vi "Select Hardware.vi"(8 "error in (no error)":errorcluster, 10 "Hardware":T4(ring), 11 "File INI.Hardware DAQ":T3) -> (0 "error out":errorcluster, 2 "#Parametros HW":T2, 3 "Reference HW":T1)   [LabVIEW 2020, in "Hardware DAQ.lvlib"]
uses:
  Hardware DAQ.lvlib
  <vilib>/Modbus/master/Modbus Master.lvclass
  <vilib>/Instr/_visa.llb/VISA Configure Serial Port (Instr).vi
  <vilib>/Modbus/master/Create Master Instance (TCP).vi
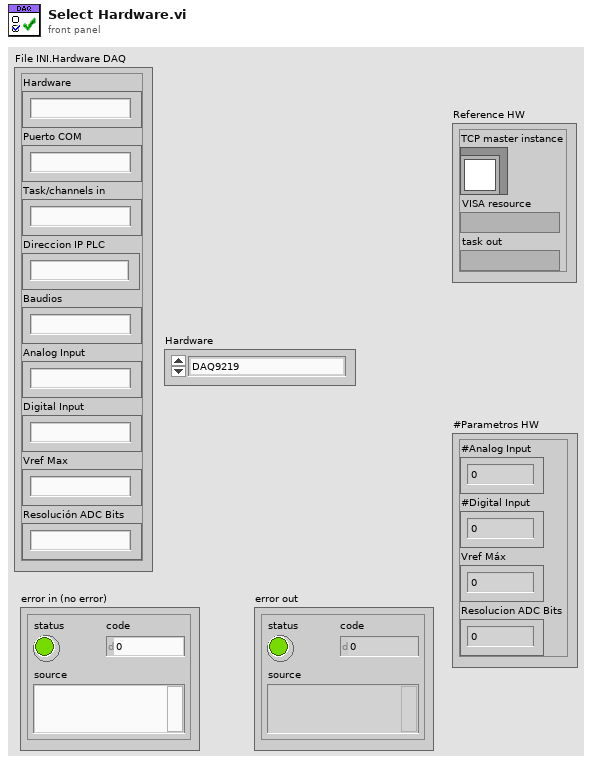
[diagram p1: front panel]
types:
  T1 = cluster{"TCP master instance":refnum<class "Modbus Master.lvclass">, "VISA resource":refnum<visa-resource-name>, "task out":refnum<k21>}
  T2 = cluster{"#Analog Input":i32, "#Digital Input":i32, "Vref Máx":i32, "Resolucion ADC Bits":i32}
  T3 = cluster{"Hardware":string, "Puerto COM":string, "Task/channels in":string, "Direccion IP PLC":string, "Baudios":string, "Analog Input":string, "Digital Input":string, "Vref Max":string, "Resolución ADC Bits":string}
  T4 = enum16{"DAQ9219", "Arduino", "Xpress Board", "PLC Logo", "Default"}
  T5 = cluster{"TCP master instance":refnum<class "Modbus Master.lvclass">, "VISA resource name out":refnum<visa-resource-name>, "task out":refnum<k21>}
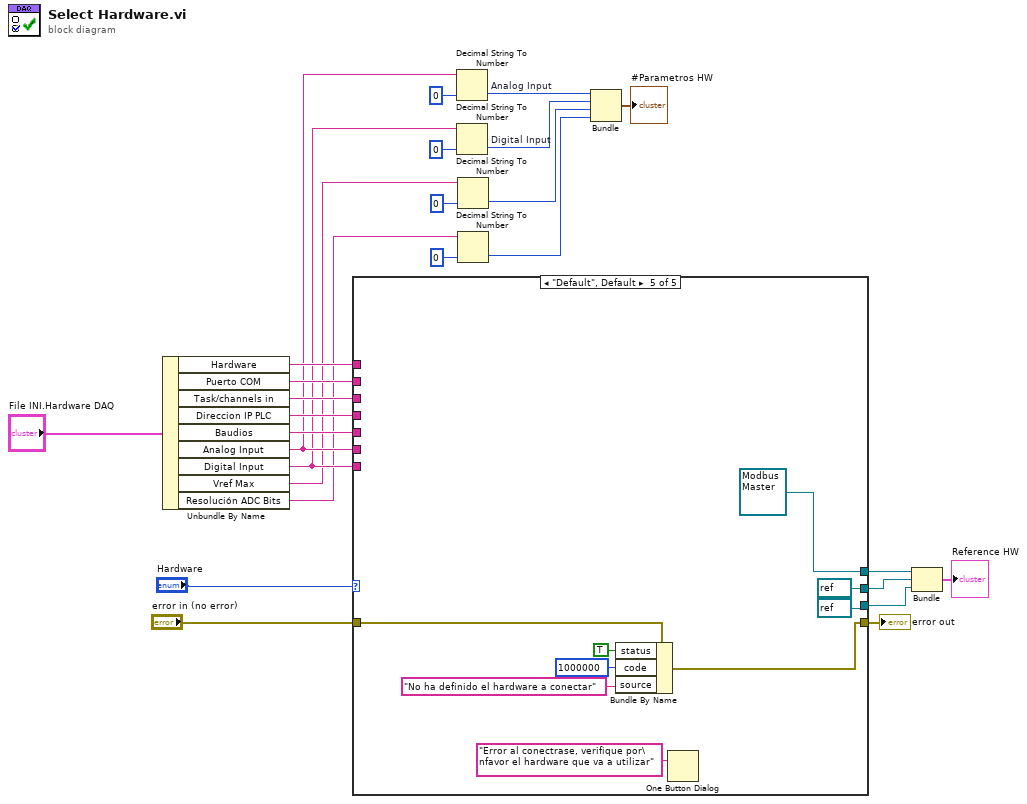
[diagram p0: block diagram]
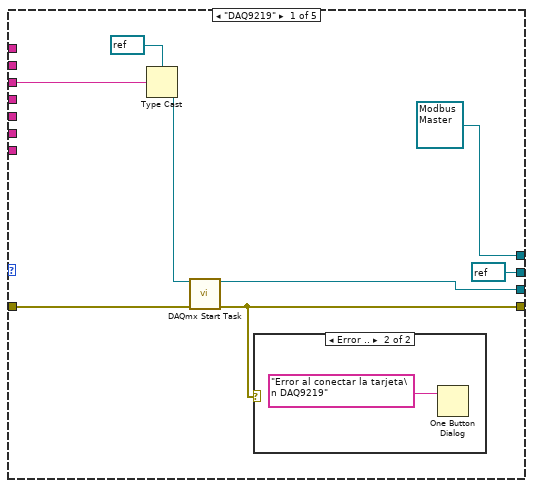
[diagram p2: hidden frame]
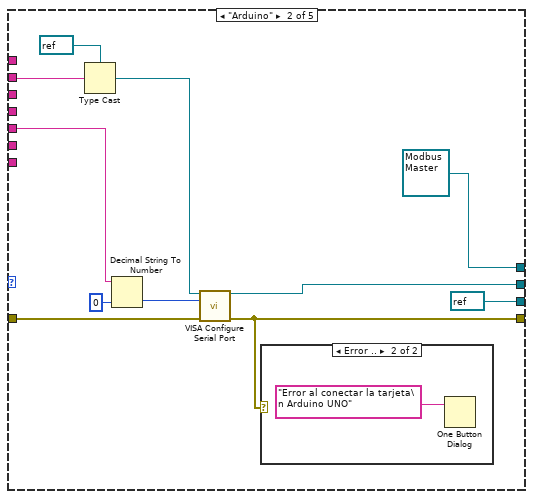
[diagram p4: hidden frame]
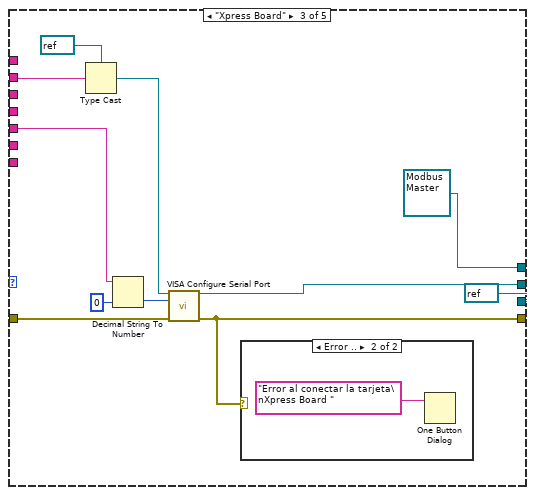
[diagram p6: hidden frame]
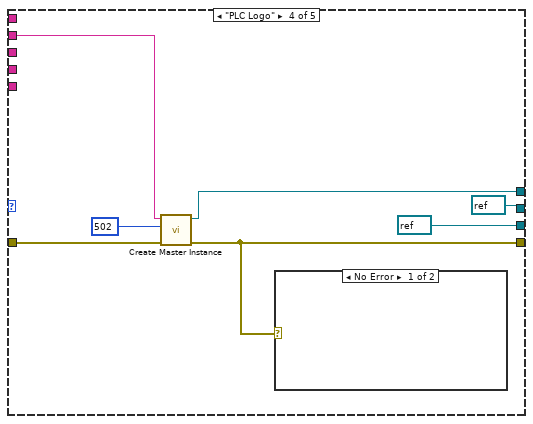
[diagram p8: hidden frame]
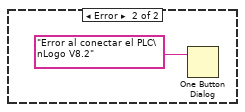
[diagram p9: hidden frame]
diagram:
  n1 = Unbundle By Name("File INI.Hardware DAQ") -> ("Hardware"=w20:string, "Puerto COM"=w21:string, "Task/channels in"=w24:string, "Direccion IP PLC"=w23:string, "Baudios"=w22:string, "Analog Input"=w19:string, "Digital Input"=w16:string, "Vref Max"=w11:string, "Resolución ADC Bits"=w10:string)
  n2 = case shown="\"Default\", Default" "Hardware" {
    tunnel: "error in (no error)" -> [w32 w44 w55 w65 w72]
    tunnel: [w27 w36 w48 w60 w70] -> w26
    tunnel: w21 -> [_ w37 w57 _ _]
    tunnel: [w31 refnum<k21> refnum ("task out") refnum<k21> refnum ("task out") refnum<k21> refnum ("task out") refnum<k21> refnum ("task out")] -> w2
    tunnel: [refnum<visa-resource-name> refnum ("VISA resource name out") w41 w52 refnum<visa-resource-name> refnum ("VISA resource name out") refnum<visa-resource-name> refnum ("VISA resource name out")] -> w3
    tunnel: w24 -> [w28 _ _ _ _]
    tunnel: w23 -> [_ _ _ w63 _]
    tunnel: w22 -> [_ w38 w49 _ _]
    tunnel: w19 -> [_ _ _ _ _]
    tunnel: w16 -> [_ _ _ _ _]
    tunnel: [refnum<class "Modbus Master.lvclass"> refnum ("TCP master instance") refnum<class "Modbus Master.lvclass"> refnum ("TCP master instance") refnum<class "Modbus Master.lvclass"> refnum ("TCP master instance") w62 refnum<class "Modbus Master.lvclass"> refnum ("TCP master instance")] -> w4
    tunnel: w20 -> [_ _ _ _ _]
    frame "DAQ9219" {
      n3 = Type Cast(type=refnum<k21> refnum ("task/channels in"), x=w28) -> (*(type *) &x=w33:refnum<k21>)
      n4 = call <vilib>:"DAQmx Start Task.vi"("task/channels in"=w33, "error in"=w32) -> ("task out"=w31:refnum<k21>, "error out"=w27:errorcluster)  [unwired: 12 in]
      n5 = case shown="Error .." w27 {
        frame No Error {
        }
        frame Error {
          n6 = One Button Dialog(message="Error al conectar la tarjeta\n DAQ9219") -> ()  [unwired: 1 in, 1 out]
        }
      }
    }
    frame "Arduino" {
      n7 = Type Cast(type=refnum<visa-resource-name> refnum ("VISA resource name"), x=w37) -> (*(type *) &x=w45:refnum<visa-resource-name>)
      n8 = Decimal String To Number(string=w38, default (0L)=u32 0 ("default (0 I32)")) -> (number=w42:u32)  [unwired: 1 in, 1 out]
      n9 = call-poly "VISA Configure Serial Port"("VISA resource name"=w45, "baud rate (9600)"=w42, "error in (no error)"=w44) -> ("VISA resource name out"=w41:refnum<visa-resource-name>, "error out"=w36:errorcluster)  [unwired: 11 in]
      n10 = case shown="Error .." w36 {
        frame No Error {
        }
        frame Error {
          n11 = One Button Dialog(message="Error al conectar la tarjeta\n Arduino UNO") -> ()  [unwired: 1 in, 1 out]
        }
      }
    }
    frame "Xpress Board" {
      n12 = Type Cast(type=refnum<visa-resource-name> refnum ("VISA resource name"), x=w57) -> (*(type *) &x=w56:refnum<visa-resource-name>)
      n13 = Decimal String To Number(string=w49, default (0L)=u32 0 ("default (0 I32)")) -> (number=w53:u32)  [unwired: 1 in, 1 out]
      n14 = call-poly "VISA Configure Serial Port"("VISA resource name"=w56, "baud rate (9600)"=w53, "error in (no error)"=w55) -> ("VISA resource name out"=w52:refnum<visa-resource-name>, "error out"=w48:errorcluster)  [unwired: 11 in]
      n15 = case shown="Error .." w48 {
        frame No Error {
        }
        frame Error {
          n16 = One Button Dialog(message="Error al conectar la tarjeta\nXpress Board ") -> ()  [unwired: 1 in, 1 out]
        }
      }
    }
    frame "PLC Logo" {
      n17 = call-poly <vilib>:"Create Master Instance.vi"("error in (no error)"=w65, "port (502)"=u16 502, "address"=w63) -> ("error out"=w60:errorcluster, "TCP master instance"=w62:refnum<class "Modbus Master.lvclass">)  [unwired: 7 in]
      n18 = case shown="No Error" w60 {
        frame No Error {
        }
        frame Error {
          n19 = One Button Dialog(message="Error al conectar el PLC\nLogo V8.2") -> ()  [unwired: 1 in, 1 out]
        }
      }
    }
    frame "Default", Default {
      n20 = Bundle By Name(cluster=w72, "status"=TRUE, "code"=1000000, "source"="No ha definido el hardware a conectar") -> (w70:errorcluster)
      n21 = One Button Dialog(message="Error al conectrase, verifique por\nfavor el hardware que va a utilizar") -> ()  [unwired: 1 in, 1 out]
    }
  }
  "error out" <- w26
  n22 = Decimal String To Number "Analog Input"(string=w19, default (0L)=0) -> (number=w9:i32)  [unwired: 1 in, 1 out]
  n23 = Decimal String To Number "Digital Input"(string=w16, default (0L)=0) -> (number=w8:i32)  [unwired: 1 in, 1 out]
  n24 = Decimal String To Number ("Analog Input")(string=w11, default (0L)=0) -> (number=w7:i32)  [unwired: 1 in, 1 out]
  n25 = Decimal String To Number ("Digital Input")(string=w10, default (0L)=0) -> (number=w6:i32)  [unwired: 1 in, 1 out]
  n26 = Bundle(w9, w8, w7, w6) -> (→"#Parametros HW":cluster{i32, i32, i32, i32})  [unwired: 1 in]
  n27 = Bundle("TCP master instance"=w4, "VISA resource name out"=w3, "task out"=w2) -> (→"Reference HW":T5)  [unwired: 1 in]
